vi "ReadWrite.Initialize.vi"(8 "error in":errorcluster, 10 "PluginAPIs":T1, 11 "Settings":T2 {"Refs" format="%.0x"}) -> (0 "error out":errorcluster, 3 "ReadWrite out":refnum<class "ReadWrite.lvclass">)   [LabVIEW 2023, in "Plugin Data Access Engine.lvlib" / "ReadWrite.lvclass"]
uses:
  ReadWrite.lvclass
  ReadWrite.lvclass/ReadWrite.ctl
  Program Files/NI/LVAddons/VS-CD-Plugin/1/Targets/win64/user.lib/PluginCore_v1.lvlibp/iPluginAPIs/iPluginAPIs.lvclass
  _PluginCore/Types/Plugin API.ctl
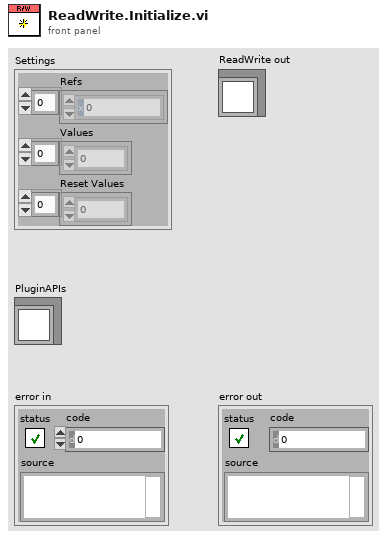
[diagram p1: front panel]
types:
  T1 = typedef "Plugin API.ctl" = refnum<class "iPluginAPIs.lvclass">
  T2 = cluster{"Refs":i32[], "Values":dbl[], "Reset Values":dbl[]}
  T3 = cluster{"read mode":enum16{"polling", "blocking"}, "write mode":enum16{"polling", "blocking"}}
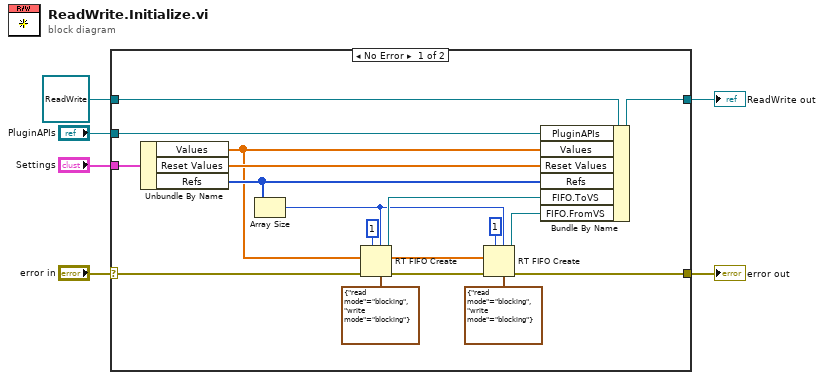
[diagram p0: block diagram]
diagram:
  n1 = case shown="No Error" "error in" {
    selector: "error in" -> [w12 w25]
    tunnel: [w17 w25] -> w6
    tunnel: refnum<class "ReadWrite.lvclass"> refnum ("ReadWrite in") -> [w14 w24]
    tunnel: [w13 w24] -> w4
    tunnel: "Settings" -> [w11 _]
    tunnel: "PluginAPIs" -> [w7 _]
    frame No Error {
      n2 = Unbundle By Name(w11) -> ("Values"=w8:dbl[], "Reset Values"=w9:dbl[], "Refs"=w10:i32[])
      n3 = Array Size(array=w10) -> (size(s)=w16:i32)
      n4 = RT FIFO Create(1:w8, 3:w12, 4:u32 1 ("size (10)"), 6:w16, 7:T3 {"read mode"=enum."blocking", "write mode"=enum."blocking"} ("r/w modes (polling,polling)")) -> (8:w22:refnum<k33>, 11:w15:errorcluster)  [unwired: 3 in, 1 out]
      n5 = RT FIFO Create(1:w8, 3:w15, 4:u32 1 ("size (10)"), 6:w16, 7:T3 {"read mode"=enum."blocking", "write mode"=enum."blocking"} ("r/w modes (polling,polling)")) -> (8:w23:refnum<k33>, 11:w17:errorcluster)  [unwired: 3 in, 1 out]
      n6 = Bundle By Name(cluster=w14, "PluginAPIs"=w7, "Values"=w8, "Reset Values"=w9, "Refs"=w10, "FIFO.ToVS"=w22, "FIFO.FromVS"=w23) -> (w13:refnum<class "ReadWrite.lvclass">)
    }
    frame Error {
    }
  }
  "error out" <- w6
  "ReadWrite out" <- w4
